vi "Anemo Receiver with Threshold.vi"() -> ()   [LabVIEW 2015]
doc: "Use this VI with the UDP Sender VI. Run this VI first.\n\nThe UDP protocol differs from TCP in that there is no error-checking with the packets of information that are sent, and thus no guarantee whatsoever that an intended recipient will actually receive a given piece of data.\n\nUDP does offer the ability to \"broadcast\" data across a network--simply specify an IP Address of all ones (255.255.255.255) to attempt to broadcast information network-wide. Keep in mind that routers and other network hardware will generally refuse to forward the broadcast beyond certain points, so the extent of the broadcast will in practice be limited."
uses:
  Anemometry/Anemometry Sub Vis/Globals/Meas_global.vi
  <vilib>/Utility/file.llb/Write To Spreadsheet File (DBL).vi
panel:
  out "Triggered":bool
  in  "Threshold":dbl=9.0
  out "speed2":dbl
  out "speed1":dbl
  out "AnemoString1":string
  in  "Port 2":u16=61557
  out "AnemoString2":string
  in  "max bytes/read":i32=548
  in  "Port":u16=61558
  in  "stop":bool
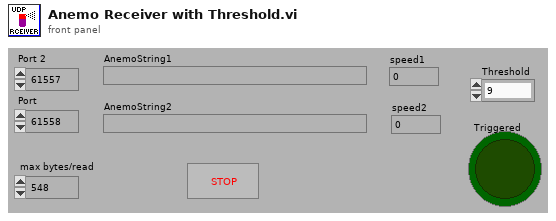
[diagram p1: front panel]
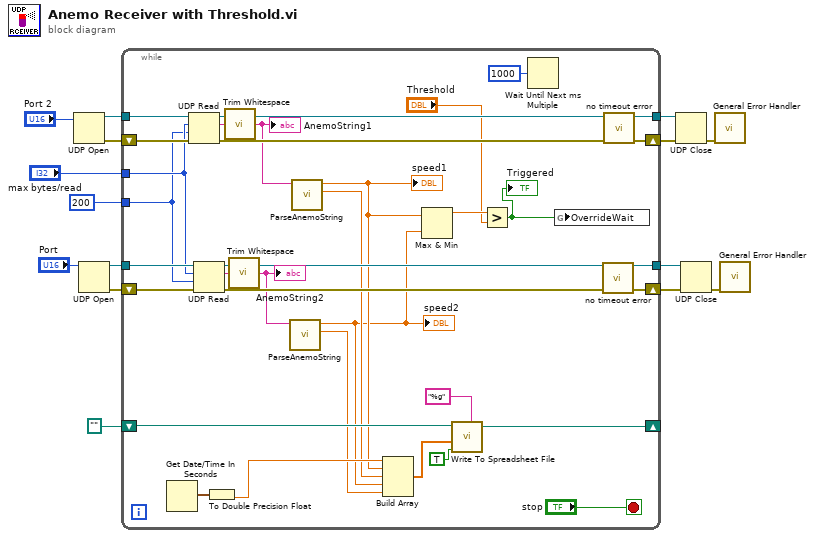
[diagram p0: block diagram]
diagram:
  n1 = UDP Open(11:"Port 2") -> (port=w4:refnum<k16>, 0:w3:errorcluster)  [unwired: 4 in, 1 out]
  n2 = UDP Open(11:"Port") -> (port=w13:refnum<k16>, 0:w14:errorcluster)  [unwired: 4 in, 1 out]
  n3 = while {
    tunnel: [w45] -> w12
    tunnel: w13 -> [w46]
    shift-left: w14 -> [w47]
    shift-right: [w43] -> w11
    tunnel: "max bytes/read" -> [w35]
    tunnel: 200 -> [w34]
    tunnel: [w38] -> w5
    tunnel: w4 -> [w37]
    shift-right: [w40] -> w6
    shift-left: w3 -> [w36]
    shift-right: [w30] -> _
    shift-left: path "" -> [w28]
    stop <- "stop" stop-if-true
    n4 = Get Date/Time In Seconds() -> (seconds since 1Jan1904=w33:timestamp)
    n5 = UDP Read(connection ID=w37, max size (548)=w35, timeout ms (25000)=w34, 8:w36) -> (data out=w31:string, error out=w39:errorcluster, 3:w38:refnum<k16>)  [unwired: 2 out]
    n6 = UDP Read(connection ID=w46, max size (548)=w35, timeout ms (25000)=w34, 8:w47) -> (data out=w32:string, error out=w44:errorcluster, 3:w45:refnum<k16>)  [unwired: 2 out]
    n7 = To Double Precision Float(number=w33) -> (double precision float=w21:dbl)
    n8 = call <vilib>:"Trim Whitespace.vi"("string"=w31) -> ("trimmed string"=w23:string)  [unwired: 1 in]
    "AnemoString1" <- w23
    n9 = call <vilib>:"Trim Whitespace.vi"("string"=w32) -> ("trimmed string"=w22:string)  [unwired: 1 in]
    "AnemoString2" <- w22
    n10 = call "ParseAnemoString.vi"("String"=w22) -> ("direction"=w17:dbl, "speed"=w18:dbl)  [unwired: 8 in, 1 out]
    "speed2" <- w18
    n11 = call "ParseAnemoString.vi"("String"=w23) -> ("direction"=w19:dbl, "speed"=w20:dbl)  [unwired: 8 in, 1 out]
    "speed1" <- w20
    n12 = Build Array(w21, w20, w19, w18, w17) -> (w16:dbl[])
    n13 = Max & Min(x=w20, y=w18) -> (max(x,y)=w26:dbl)  [unwired: 1 out]
    n14 = call-poly <vilib>:"Write To Spreadsheet File.vi"("format (%.3f)"="%g", "append to file? (new file:F)"=TRUE, "1D data"=w16, "file path (dialog if empty)"=w28) -> ("new file path (Not A Path if cancelled)"=w30:path)  [unwired: 4 in]
    n15 = Greater?(x=w26, y="Threshold") -> (0:w24:bool)
    "Triggered" <- w24
    n16 = Wait Until Next ms Multiple(millisecond multiple=u32 1000) -> ()  [unwired: 1 out]
    n17 = global write "Meas_global.vi" "OverrideWait"(w24) -> ()
    n18 = call "no timeout error.vi"("error in (no error)"=w44) -> ("error out"=w43:errorcluster)
    n19 = call "no timeout error.vi"("error in (no error)"=w39) -> ("error out"=w40:errorcluster)
  }
  n20 = UDP Close(connection ID=w5, 8:w6) -> (error out=w7:errorcluster)  [unwired: 1 out]
  n21 = UDP Close(connection ID=w12, 8:w11) -> (error out=w10:errorcluster)  [unwired: 1 out]
  n22 = call <vilib>:"General Error Handler.vi"("error in (no error)"=w7) -> ()  [unwired: 10 in, 5 out]
  n23 = call <vilib>:"General Error Handler.vi"("error in (no error)"=w10) -> ()  [unwired: 10 in, 5 out]
